vi "SamplingInfoToTimeout.vi"(7 "error in":errorcluster, 9 "sampling info":T1={"Fs"=10000.0, "#s"=1000}) -> (0 "error out":errorcluster, 2 "timeout (ms)":i32=100)   [LabVIEW 2016, in "DAQ.lvclass"]
uses:
  DAQ.lvclass
  Typedefs/DAQ_SamplingInfo.ctl
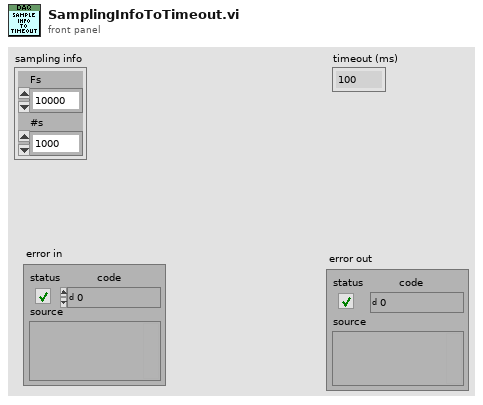
[diagram p1: front panel]
types:
  T1 = typedef "DAQ.lvclass/DAQ_SamplingInfo.ctl" = cluster{"Fs":dbl, "#s":i32}
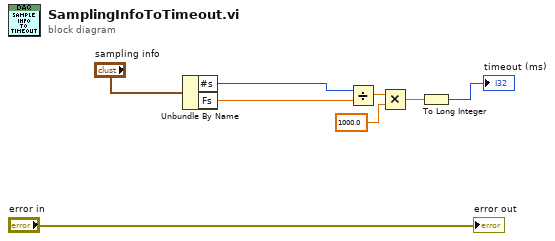
[diagram p0: block diagram]
diagram:
  n1 = Unbundle By Name("sampling info") -> ("#s"=w2:i32, "Fs"=w3:dbl)
  n2 = Divide(x=w2, y=w3) -> (x/y=w6:dbl)
  n3 = Multiply(x=w6, y=1000.0) -> (x*y=w8:dbl)
  n4 = To Long Integer(number=w8) -> (32bit integer=→"timeout (ms)":i32)
  "error out" <- "error in"
